vi "SiosIfmSetOption.vi"(1 "Option":i32(ring) items=["IFM_OPTION_DEBUGFILES"=1, "IFM_OPTION_POLLSELF"=2, "IFM_OPTION_BLOCKONCLOSE"=3, "IFM_OPTION_BOOTLOADER"=4, "IFM_OPTION_BEAMBREAK"=5], 2 "Param 1":i32) -> (0 "Success":i32)   [LabVIEW 2009]
uses:
  siosifm.dll
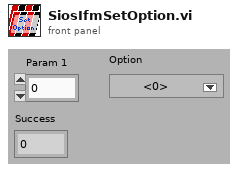
[diagram p1: front panel]
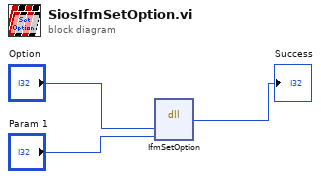
[diagram p0: block diagram]
diagram:
  n1 = dll-call lib="C:/WORK/Artem/RE-10/SIOS_IfmDLL/siosifm.dll" fn="IfmSetOption"("option"="Option", "param1"="Param 1") -> ("success"=→"Success":i32)  [unwired: 5 in, 2 out]
